vi "属性节点.vi"() -> ()   [LabVIEW 2018]
panel:
  out "布尔 2":bool
  in  "停止":bool
  out "布尔":bool
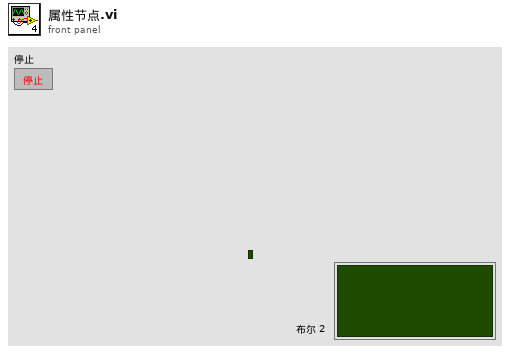
[diagram p1: front panel]
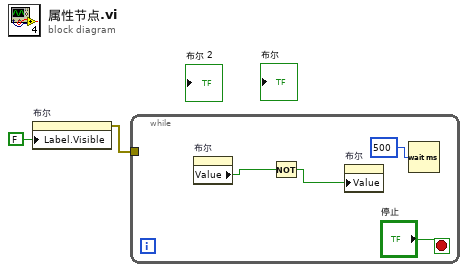
[diagram p0: block diagram]
diagram:
  n1 = property on="布尔" class="Bool (严格)"("Label.Visible"=FALSE ("标签.可见")) -> (error out=w1:errorcluster)  [unwired: 2 in, 1 out]
  n2 = while {
    tunnel: w1 -> [_]
    stop <- "停止" stop-if-true
    n3 = property on="布尔" class="Bool (严格)"() -> ("Value"=w6:bool)  [unwired: 2 in, 2 out]
    n4 = Not(x=w6) -> (.not. x?=w5:bool)
    n5 = property on="布尔" class="Bool (严格)"("Value"=w5) -> ()  [unwired: 2 in, 2 out]
    n6 = Wait (ms)(milliseconds to wait=u32 500 ("毫秒计时值")) -> ()  [unwired: 1 out]
  }
